vi "notes_to_xml.vi"(11 "Notes (in)":string) -> (3 "Notes":string)   [LabVIEW 2012]
doc: "This .vi just passes the notes through. The add_xml_headers.xml will add the <Notes></Notes> tags.\n\nMTL 2012 Dec 31"
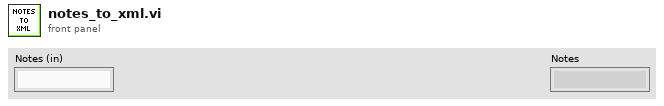
[diagram p1: front panel]
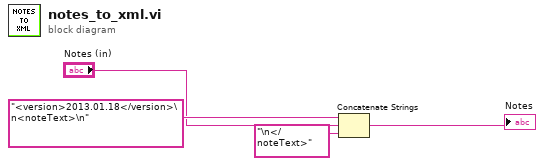
[diagram p0: block diagram]
diagram:
  n1 = Concatenate Strings("<version>2013.01.18</version>\n<noteText>\n" ("string"), "Notes (in)", "\n</noteText>" ("string")) -> (→"Notes":string)
